vi "BS find all the buoys.vi"(0 "Image Src":T1, 1 "error in":errorcluster) -> (2 "Buoy Array":cluster{i16, i16}[](array[cluster]), 3 "Buoys found?":bool, 4 "error out":errorcluster)   [LabVIEW 2012]
doc: "This VI finds all the buoys and places there location into a 2D array. A valid flag is posted if completed."
uses:
  <vilib>/vision/Image Controls.llb/IMAQ Image.ctl
  <vilib>/vision/NI_Vision_Development_Module.lvlib
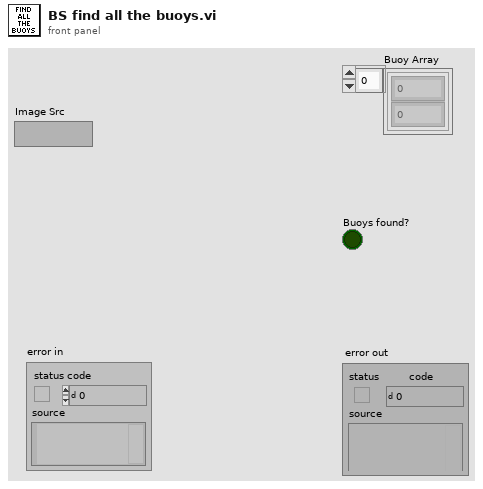
[diagram p1: front panel]
types:
  T1 = typedef "IMAQ Image.ctl" = refnum<image>
  T2 = enum32{"AutoM", "Close", "Dilate", "Erode", "Gradient", "Gradient in", "Gradient out", "HitMiss", "Open", "PClose", "POpen", "Thick", "Thin"}
  T3 = cluster{"Position":cluster{"x":sgl, "y":sgl}, "Angle":sgl, "Scale":sgl, "Score":sgl, "Bounding Box":cluster{"x":sgl, "y":sgl}[]}[]
  T4 = cluster{"Position":cluster{"x":sgl, "y":sgl}, "Angle":sgl, "Scale":sgl, "Score":sgl, "Bounding Box":cluster{"x":sgl, "y":sgl}[]}
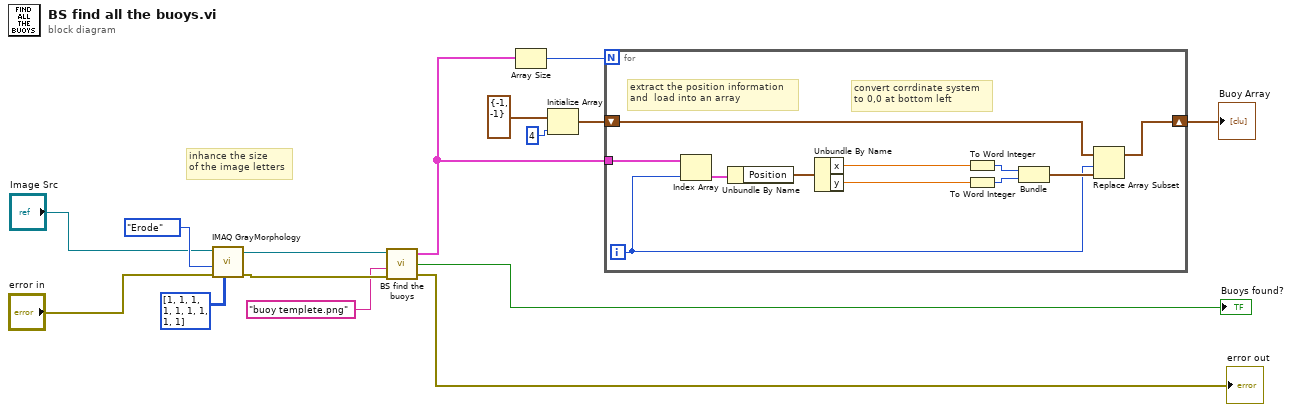
[diagram p0: block diagram]
diagram:
  # "inhance the size \nof the image letters"
  n1 = call "IMAQ GrayMorphology"("Structuring Element"=i32[][] [[1, 1, 1], [1, 1, 1], [1, 1, 1]] ("Structuring Element (Gray Morphology 1)"), "error in (no error)"="error in", "Operation"=T2."Erode" ("Operation (Gray Morphology 1)"), "Image Src"="Image Src") -> ("error out"=w10:errorcluster, "Image Dst Out"=w11:T1)  [unwired: 3 in, 3 out]
  n2 = call "BS find the buoys.vi"("Image Path"=w11, "templete path"="buoy templete.png", "error in"=w10) -> ("Matches"=w6:T3, "Valid?"=→"Buoys found?":bool, "error out"=→"error out":errorcluster)  [unwired: 2 in]
  n3 = Array Size(array=w6) -> (size(s)=w5:i32)
  n4 = Initialize Array(cluster{i16, i16} {-1, -1} ("buoy cluster"), 4 ("dimension size")) -> (w2:cluster{i16, i16}[])
  n5 = for {
    N: w5 -> [_]
    tunnel: w6 -> [w25]
    shift-right: [w17] -> w1
    shift-left: w2 -> [w20]
    i -> [w18]
    # "convert corrdinate system\nto 0,0 at bottom left"
    # "extract the position information\nand  load into an array"
    n6 = Index Array(array=w25, index=w18) -> (element=w26:T4)
    n7 = Unbundle By Name(w26) -> ("Position"=w23:cluster{"x":sgl, "y":sgl})
    n8 = Unbundle By Name(w23) -> ("x"=w24:sgl, "y"=w16:sgl)
    n9 = To Word Integer(number=w24) -> (16bit integer=w22:i16)
    n10 = To Word Integer(number=w16) -> (16bit integer=w21:i16)
    n11 = Bundle(w22, w21) -> (w19:cluster{i16, i16})  [unwired: 1 in]
    n12 = Replace Array Subset(array=w20, new element=w19, index=w18) -> (w17:cluster{i16, i16}[])
  }
  "Buoy Array" <- w1
